vi "GetTerms4.vi"(0 "XRef":T11, 1 "State In":T10) -> (14 "Terms":T2, 15 "Fatal Error Out":T1)   [LabVIEW 2015, in "Get Object Parameters.xnode"]
uses:
  Get Object Parameters.xnode
  <vilib>/XNodeSupport/XNodeXNodeRef.ctl
  State.ctl
  <vilib>/XNodeSupport/XNodeTerm4Array.ctl
  <vilib>/XNodeSupport/XNodeTerm4.ctl
  <vilib>/XNodeSupport/XNodeString.ctl
  <vilib>/XNodeSupport/XNodeVariant.ctl
  <vilib>/XNodeSupport/XNodeRect32.ctl
  <vilib>/XNodeSupport/XNodeInt.ctl
  <vilib>/XNodeSupport/XNodeBool.ctl
  <vilib>/XNodeSupport/XNodeTermDirection.ctl
  <vilib>/XNodeSupport/XNodeErrorCluster.ctl
  JSON Object.lvclass
  JSON Datatype/JSON Null.lvclass
  JSON String/JSON String.lvclass
  JSON Numeric/JSON Numeric.lvclass
  JSON Boolean/JSON Boolean.lvclass
  JSON Array/JSON Array.lvclass
  dimensions.vi
  <vilib>/XNodeSupport/NI_XNodeSupport.lvlib
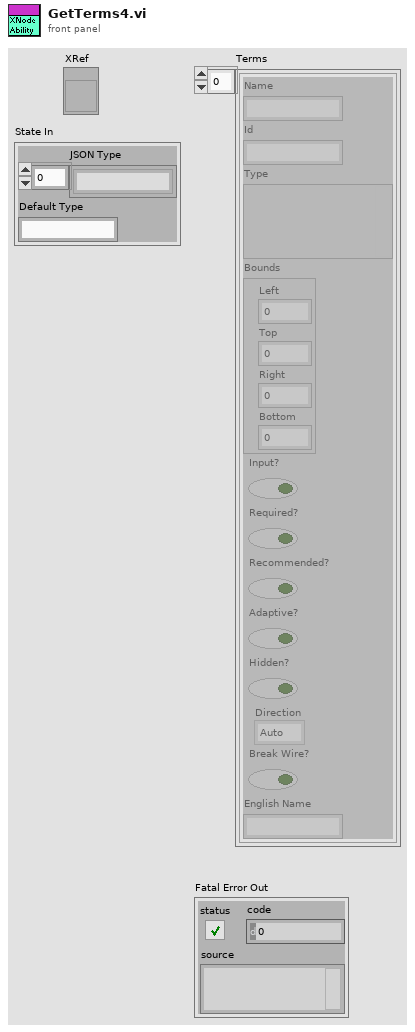
[diagram p1: front panel]
types:
  T1 = typedef "NI_XNodeSupport.lvlib/XNodeErrorCluster.ctl" = errorcluster
  T2 = typedef "NI_XNodeSupport.lvlib/XNodeTerm4Array.ctl" = T3[]
  T3 = typedef "NI_XNodeSupport.lvlib/XNodeTerm4.ctl" = cluster{"Name":T4, "Id":T4, "Type":T5, "Bounds":T6, "Input?":T8, "Required?":T8, "Recommended?":T8, "Adaptive?":T8, "Hidden?":T8, "Direction":T9, "Break Wire?":T8, "English Name":T4}
  T4 = typedef "NI_XNodeSupport.lvlib/XNodeString.ctl" = string
  T5 = typedef "NI_XNodeSupport.lvlib/XNodeVariant.ctl" = variant
  T6 = typedef "NI_XNodeSupport.lvlib/XNodeRect32.ctl" = cluster{"Left":T7, "Top":T7, "Right":T7, "Bottom":T7}
  T7 = typedef "NI_XNodeSupport.lvlib/XNodeInt.ctl" = i32
  T8 = typedef "NI_XNodeSupport.lvlib/XNodeBool.ctl" = bool
  T9 = typedef "NI_XNodeSupport.lvlib/XNodeTermDirection.ctl" = enum32{"Auto", "Up", "Down", "Left", "Right", "Center"}
  T10 = typedef "Get Object Parameters.xnode/State.ctl" = cluster{"JSON Type":string[], "Default Type":string}
  T11 = typedef "NI_XNodeSupport.lvlib/XNodeXNodeRef.ctl" = refnum<vi>
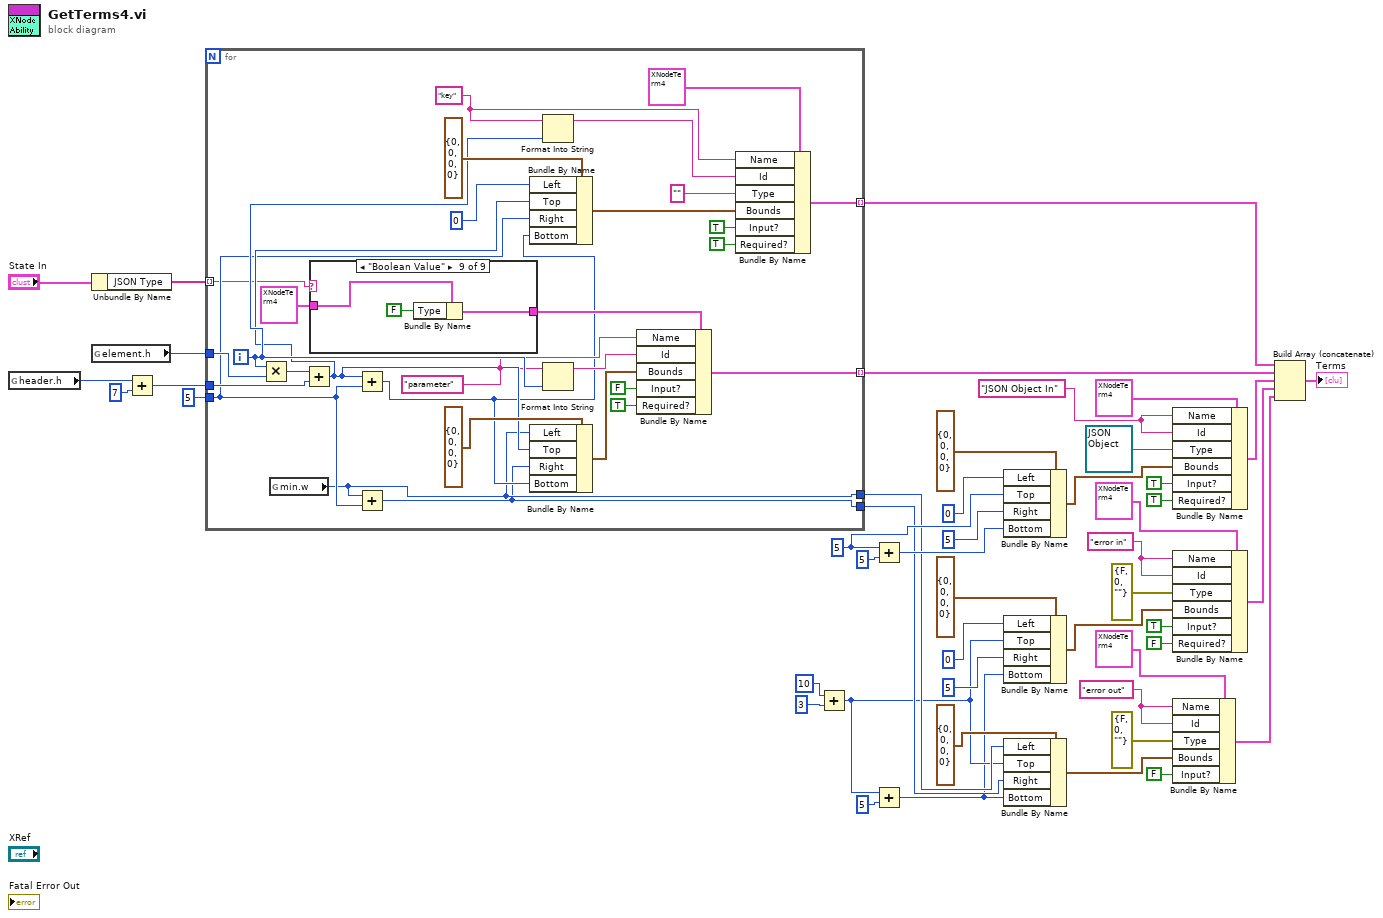
[diagram p0: block diagram]
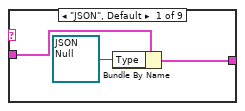
[diagram p2: hidden frame]
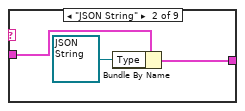
[diagram p3: hidden frame]
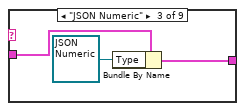
[diagram p4: hidden frame]
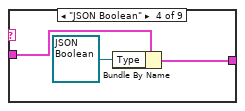
[diagram p5: hidden frame]
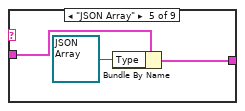
[diagram p6: hidden frame]
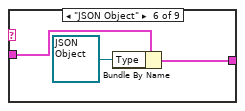
[diagram p7: hidden frame]
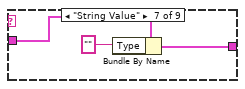
[diagram p8: hidden frame]
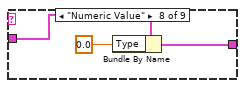
[diagram p9: hidden frame]
diagram:
  w8 = T4 "error out" ("Name")
  w20 = T4 "error in" ("Name")
  w30 = T7 5 ("Top")
  w36 = T4 "JSON Object In" ("Name")
  n1 = global read "dimensions.vi" "header.h"() -> (w44:i16)
  n2 = Unbundle By Name("State In") -> ("JSON Type"=w25:string[])
  n3 = global read "dimensions.vi" "element.h"() -> (w46:i16)
  n4 = Add(x=w44, y=7) -> (x+y=w42:i32)
  n5 = for {
    tunnel: w46 -> [w70]
    tunnel: w42 -> [w67]
    tunnel: T7 5 ("Right") -> [w59]
    tunnel: [w56] -> w27 mode=indexing
    tunnel: [w55] -> w26 mode=indexing
    tunnel: w25 -> [w54] mode=indexing
    tunnel: [w50] -> w5
    tunnel: [w49] -> w4
    i -> [w61]
    w57 = "parameter" ("initial string")
    w58 = "key" ("initial string")
    n6 = Multiply(x=w61, y=w70) -> (x*y=w68:i32)
    n7 = global read "dimensions.vi" "min.w"() -> (w50:i32)
    n8 = Add(x=w68, y=w67) -> (x+y=w60:i32)
    n9 = case shown="\"Boolean Value\"" w54 {
      tunnel: T3 {"Name"="", "Id"="", "Type"=variant, "Bounds"={"Left"=0, "Top"=0, "Right"=0, "Bottom"=0}, "Input?"=FALSE, "Required?"=FALSE, "Recommended?"=FALSE, "Adaptive?"=FALSE, "Hidden?"=FALSE, "Direction"=enum."Auto", "Break Wire?"=FALSE, "English Name"=""} ("Term 4") -> [w79 w82 w85 w88 w91 w94 w97 w100 w103]
      tunnel: [w77 w80 w83 w86 w89 w92 w96 w99 w102] -> w52
      frame "JSON", Default {
        n10 = Bundle By Name(cluster=w79, "Type"=refnum<class "JSON Null.lvclass"> refnum ("LVJSON.lvlib:JSON Null.lvclass")) -> (w77:T3)
      }
      frame "JSON String" {
        n11 = Bundle By Name(cluster=w82, "Type"=refnum<class "JSON String.lvclass"> refnum ("LVJSON.lvlib:JSON String.lvclass")) -> (w80:T3)
      }
      frame "JSON Numeric" {
        n12 = Bundle By Name(cluster=w85, "Type"=refnum<class "JSON Numeric.lvclass"> refnum ("LVJSON.lvlib:JSON Numeric.lvclass")) -> (w83:T3)
      }
      frame "JSON Boolean" {
        n13 = Bundle By Name(cluster=w88, "Type"=refnum<class "JSON Boolean.lvclass"> refnum ("LVJSON.lvlib:JSON Boolean.lvclass")) -> (w86:T3)
      }
      frame "JSON Array" {
        n14 = Bundle By Name(cluster=w91, "Type"=refnum<class "JSON Array.lvclass"> refnum ("LVJSON.lvlib:JSON Array.lvclass")) -> (w89:T3)
      }
      frame "JSON Object" {
        n15 = Bundle By Name(cluster=w94, "Type"=refnum<class "JSON Object.lvclass"> refnum ("LVJSON.lvlib:JSON Object.lvclass")) -> (w92:T3)
      }
      frame "String Value" {
        n16 = Bundle By Name(cluster=w97, "Type"="" ("initial string")) -> (w96:T3)
      }
      frame "Numeric Value" {
        n17 = Bundle By Name(cluster=w100, "Type"=0.0) -> (w99:T3)
      }
      frame "Boolean Value" {
        n18 = Bundle By Name(cluster=w103, "Type"=FALSE) -> (w102:T3)
      }
    }
    n19 = Add(x=w60, y=w59) -> (x+y=w51:T7)
    n20 = Add(x=w50, y=w59) -> (x+y=w49:T7)
    n21 = Bundle By Name(cluster=T6 {"Left"=0, "Top"=0, "Right"=0, "Bottom"=0} ("Bounds"), "Left"=T7 0, "Top"=w60, "Right"=w59, "Bottom"=w51) -> (w69:T6)
    n22 = Bundle By Name(cluster=T6 {"Left"=0, "Top"=0, "Right"=0, "Bottom"=0} ("Bounds"), "Left"=w50, "Top"=w60, "Right"=w49, "Bottom"=w51) -> (w66:T6)
    n23 = Format Into String(initial string=w58, w61) -> (resulting string=w75:string)  [unwired: 2 in, 1 out]
    n24 = Format Into String(initial string=w57, w61) -> (resulting string=w62:string)  [unwired: 2 in, 1 out]
    n25 = Bundle By Name(cluster=w52, "Name"=w57, "Id"=w62, "Bounds"=w66, "Input?"=T8 FALSE, "Required?"=T8 TRUE) -> (w56:T3)
    n26 = Bundle By Name(cluster=T3 {"Name"="", "Id"="", "Type"=variant, "Bounds"={"Left"=0, "Top"=0, "Right"=0, "Bottom"=0}, "Input?"=FALSE, "Required?"=FALSE, "Recommended?"=FALSE, "Adaptive?"=FALSE, "Hidden?"=FALSE, "Direction"=enum."Auto", "Break Wire?"=FALSE, "English Name"=""} ("Term 4"), "Name"=w58, "Id"=w75, "Type"="" ("initial string"), "Bounds"=w69, "Input?"=T8 TRUE, "Required?"=T8 TRUE) -> (w55:T3)
  }
  n27 = Add(x=T7 10, y=T7 3) -> (x+y=w3:T7)
  n28 = Add(x=w30, y=T7 5) -> (x+y=w28:T7)
  n29 = Add(x=w3, y=T7 5) -> (x+y=w2:T7)
  n30 = Bundle By Name(cluster=T6 {"Left"=0, "Top"=0, "Right"=0, "Bottom"=0} ("Bounds"), "Left"=T7 0, "Top"=w30, "Right"=T7 5, "Bottom"=w28) -> (w37:T6)
  n31 = Bundle By Name(cluster=T6 {"Left"=0, "Top"=0, "Right"=0, "Bottom"=0} ("Bounds"), "Left"=T7 0, "Top"=w3, "Right"=T7 5, "Bottom"=w2) -> (w19:T6)
  n32 = Bundle By Name(cluster=T6 {"Left"=0, "Top"=0, "Right"=0, "Bottom"=0} ("Bounds"), "Left"=w5, "Top"=w3, "Right"=w4, "Bottom"=w2) -> (w9:T6)
  n33 = Bundle By Name(cluster=T3 {"Name"="", "Id"="", "Type"=variant, "Bounds"={"Left"=0, "Top"=0, "Right"=0, "Bottom"=0}, "Input?"=FALSE, "Required?"=FALSE, "Recommended?"=FALSE, "Adaptive?"=FALSE, "Hidden?"=FALSE, "Direction"=enum."Auto", "Break Wire?"=FALSE, "English Name"=""} ("Term 4"), "Name"=w36, "Id"=w36, "Type"=refnum<class "JSON Object.lvclass"> refnum ("LVJSON.lvlib:JSON Object.lvclass"), "Bounds"=w37, "Input?"=T8 TRUE, "Required?"=T8 TRUE) -> (w32:T3)
  n34 = Bundle By Name(cluster=T3 {"Name"="", "Id"="", "Type"=variant, "Bounds"={"Left"=0, "Top"=0, "Right"=0, "Bottom"=0}, "Input?"=FALSE, "Required?"=FALSE, "Recommended?"=FALSE, "Adaptive?"=FALSE, "Hidden?"=FALSE, "Direction"=enum."Auto", "Break Wire?"=FALSE, "English Name"=""} ("Term 4"), "Name"=w20, "Id"=w20, "Type"=errorcluster {"status"=FALSE, "code"=0, "source"=""} ("error constant"), "Bounds"=w19, "Input?"=T8 TRUE, "Required?"=T8 FALSE) -> (w13:T3)
  n35 = Bundle By Name(cluster=T3 {"Name"="", "Id"="", "Type"=variant, "Bounds"={"Left"=0, "Top"=0, "Right"=0, "Bottom"=0}, "Input?"=FALSE, "Required?"=FALSE, "Recommended?"=FALSE, "Adaptive?"=FALSE, "Hidden?"=FALSE, "Direction"=enum."Auto", "Break Wire?"=FALSE, "English Name"=""} ("Term 4"), "Name"=w8, "Id"=w8, "Type"=errorcluster {"status"=FALSE, "code"=0, "source"=""} ("error constant"), "Bounds"=w9, "Input?"=T8 FALSE) -> (w6:T3)
  n36 = Build Array (concatenate)(w26, w27, w32, w13, w6) -> (→"Terms":T3[])
